vi "Draw Border On Active Graphic.vi"(8 "error in (no error)":errorcluster, 11 "Canvas in":refnum<class "Canvas.lvclass">) -> (0 "error out":errorcluster, 3 "Canvas out":refnum<class "Canvas.lvclass">)   [LabVIEW 2015, in "Canvas.lvclass"]
uses:
  Canvas.lvclass
  Canvas.lvclass/Canvas.ctl
  Graphic/Graphic.lvclass/Graphic.ctl
  Scalable Border/Scalable Border.lvclass
  Graphic/Graphic.lvclass
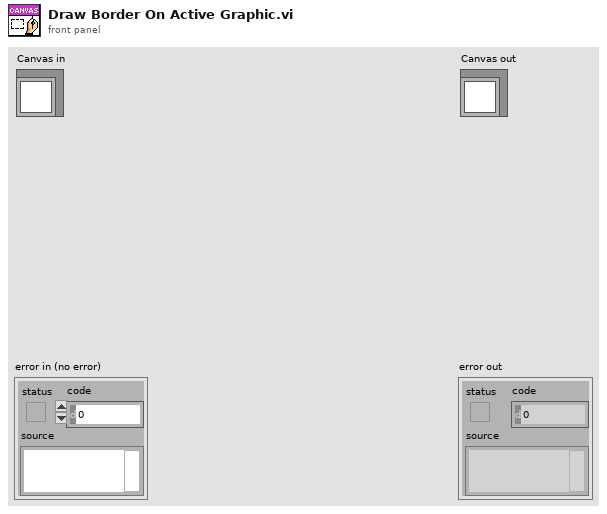
[diagram p1: front panel]
types:
  T1 = typedef "Graphic.lvclass/Style.ctl" = cluster{"Color":u32, "Pen":cluster{"Width":u16, "Style":enum32{"Solid", "Dash", "Dot", "DashDot", "DashDotDot"}}}
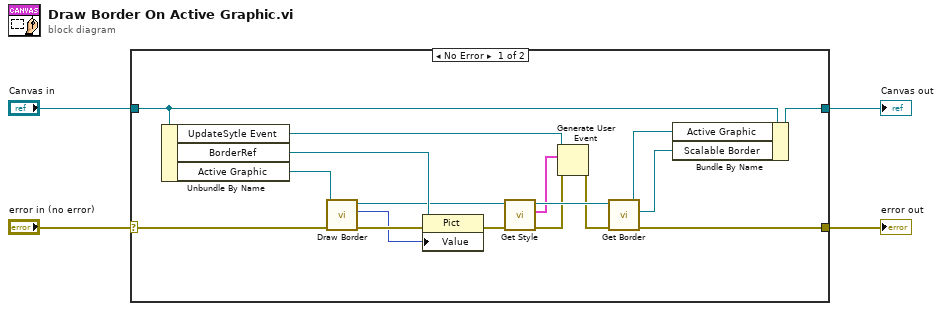
[diagram p0: block diagram]
diagram:
  n1 = case shown="No Error" "error in (no error)" {
    selector: "error in (no error)" -> [w17 w23]
    tunnel: [w13 w23] -> w3
    tunnel: [w16 w22] -> w1
    tunnel: "Canvas in" -> [w21 w22]
    frame No Error {
      n2 = Unbundle By Name(w21) -> ("UpdateSytle Event"=w8:refnum<user-event>, "BorderRef"=w20:refnum<vi>, "Active Graphic"=w12:refnum<class "Graphic.lvclass">)
      n3 = call-dynamic "Draw Border.vi"("error in (no error)"=w17, "Graphic in"=w12) -> ("error out"=w19:errorcluster, "Picture out"=w18:picture, "Graphic out"=w10:refnum<class "Graphic.lvclass">)  [unwired: 7 in]
      n4 = property class="Pict"(reference=w20, error in=w19, "Value"=w18) -> (error out=w14:errorcluster)  [unwired: 1 out]
      n5 = call "Get Style.vi"("error in (no error)"=w14, "Graphic in"=w10) -> ("error out"=w7:errorcluster, "Style"=w5:T1, "Graphic out"=w9:refnum<class "Graphic.lvclass">)  [unwired: 7 in]
      n6 = Generate User Event(user event=w8, event data cluster=w5, error in=w7) -> (error out=w6:errorcluster)  [unwired: 1 in, 1 out]
      n7 = call "Get Border.vi"("error in (no error)"=w6, "Graphic in"=w9) -> ("error out"=w13:errorcluster, "Scalable Border.lvclass"=w11:refnum<class "Scalable Border.lvclass">, "Graphic out"=w15:refnum<class "Graphic.lvclass">)  [unwired: 7 in]
      n8 = Bundle By Name(cluster=w21, "Active Graphic"=w15, "Scalable Border"=w11) -> (w16:refnum<class "Canvas.lvclass">)
    }
    frame Error {
    }
  }
  "error out" <- w3
  "Canvas out" <- w1
